vi "Status ConvBox.vi"(8 "error in (no error)":errorcluster, 11 "VISA resource name":refnum<visa-resource-name>) -> (0 "error out":errorcluster, 1 "GPIB error":i16, 2 "ibsta":T1, 3 "VISA resource out":refnum<visa-resource-name>)   [LabVIEW 2019, in "Localhost Protocols.lvlib" / "RS-xxx to GPIB ConvBox.lvclass"]
uses:
  RS-xxx to GPIB ConvBox.lvclass
  <vilib>/Instr/_visa.llb/GPIB Status Boolean Array.ctl
  <vilib>/Instr/_visa.llb/VISA Flush IO Buffer Mask.ctl
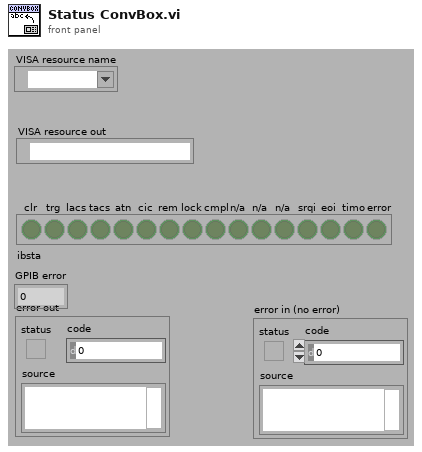
[diagram p1: front panel]
types:
  T1 = typedef "GPIB Status Boolean Array.ctl" = bool[]
  T2 = typedef "VISA Flush IO Buffer Mask.ctl" = u16
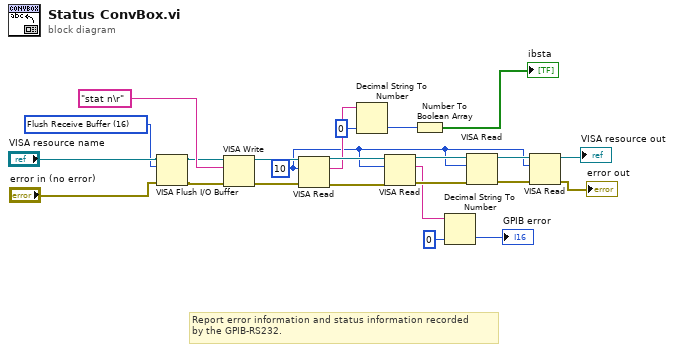
[diagram p0: block diagram]
diagram:
  w4 = T2 16 items=["Flush Receive Buffer"=16, "Write Transmit Buffer to Device"=32, "Flush Receive Buffer (No I/O)"=64, "Flush Transmit Buffer"=128] ("Mask")
  w9 = u32 10 ("byte count")
  # "Report error information and status information recorded \nby the GPIB-RS232."
  n1 = VISA Flush I/O Buffer(VISA resource name="VISA resource name", mask (16)=w4, error in (no error)="error in (no error)") -> (VISA resource name out=w7:refnum<visa-resource-name>, error out=w6:errorcluster)
  n2 = VISA Write(VISA resource name=w7, write buffer="stat n\r", error in (no error)=w6) -> (VISA resource name out=w18:refnum<visa-resource-name>, error out=w23:errorcluster)  [unwired: 1 out]
  n3 = VISA Read(VISA resource name=w18, byte count=w9, error in (no error)=w23) -> (VISA resource name out=w19:refnum<visa-resource-name>, read buffer=w17:string, error out=w22:errorcluster)  [unwired: 1 out]
  n4 = Decimal String To Number(string=w17, default (0L)=i16 0 ("default (0 I32)")) -> (number=w15:i16)  [unwired: 1 in, 1 out]
  n5 = VISA Read(VISA resource name=w19, byte count=w9, error in (no error)=w22) -> (VISA resource name out=w20:refnum<visa-resource-name>, read buffer=w2:string, error out=w21:errorcluster)  [unwired: 1 out]
  n6 = Number To Boolean Array(number=w15) -> (Boolean array=→"ibsta":bool[])
  n7 = Decimal String To Number(string=w2, default (0L)=i16 0 ("default (0 I32)")) -> (number=→"GPIB error":i16)  [unwired: 1 in, 1 out]
  n8 = VISA Read(VISA resource name=w20, byte count=w9, error in (no error)=w21) -> (VISA resource name out=w12:refnum<visa-resource-name>, error out=w13:errorcluster)  [unwired: 2 out]
  n9 = VISA Read(VISA resource name=w12, byte count=w9, error in (no error)=w13) -> (VISA resource name out=→"VISA resource out":refnum<visa-resource-name>, error out=→"error out":errorcluster)  [unwired: 2 out]
